vi "ExamplePIDDrive.vi"() -> ()   [LabVIEW 2016]
uses:
  <vilib>/addons/control/pid/pid.llb/PID (DBL).vi
  <vilib>/addons/control/pid/NI_PID_pid.lvlib
panel:
  in  "PID Segments (1-500)":dbl=1.0
  in  "Limit of Orientation Change":dbl=1.0
  in  "Absolute Theta Final":dbl
  in  "Absolute Theta initial":dbl
  in  "Y":dbl[](array[numeric])
  in  "X":dbl[](array[numeric])
  out "output 2":dbl format="%.2f"
  out "output":dbl format="%.2f"
  in  "Steer Range":cluster{"output high":dbl, "output low":dbl}={"output high"=100.0, "output low"=-100.0} {"output low" format="%.2f"; "output high" format="%.2f"}
  in  "PID Steer gains":T1={"proportional gain (Kc)"=1.0, "integral time (Ti, min)"=0.01, "derivative time (Td, min)"=0.0} {"derivative time (Td, min)" format="%.3f"; "integral time (Ti, min)" format="%.3f"; "proportional gain (Kc)" format="%.3f"}
  in  "Speed Range":cluster{"output high":dbl, "output low":dbl}={"output high"=100.0, "output low"=-100.0} {"output low" format="%.2f"; "output high" format="%.2f"}
  in  "PID Speed gains":T1={"proportional gain (Kc)"=1.0, "integral time (Ti, min)"=0.01, "derivative time (Td, min)"=0.0} {"derivative time (Td, min)" format="%.3f"; "integral time (Ti, min)" format="%.3f"; "proportional gain (Kc)" format="%.3f"}
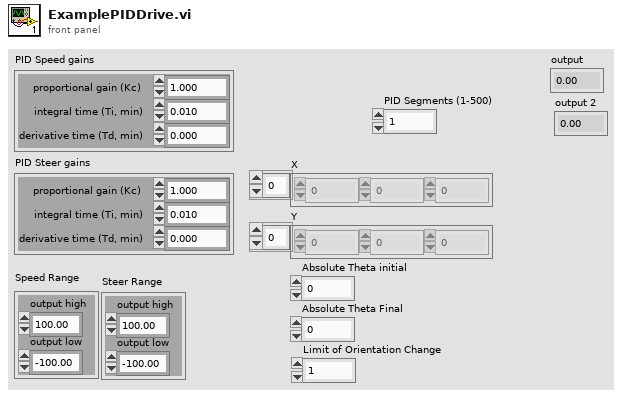
[diagram p1: front panel]
types:
  T1 = cluster{"proportional gain (Kc)":dbl, "integral time (Ti, min)":dbl, "derivative time (Td, min)":dbl}
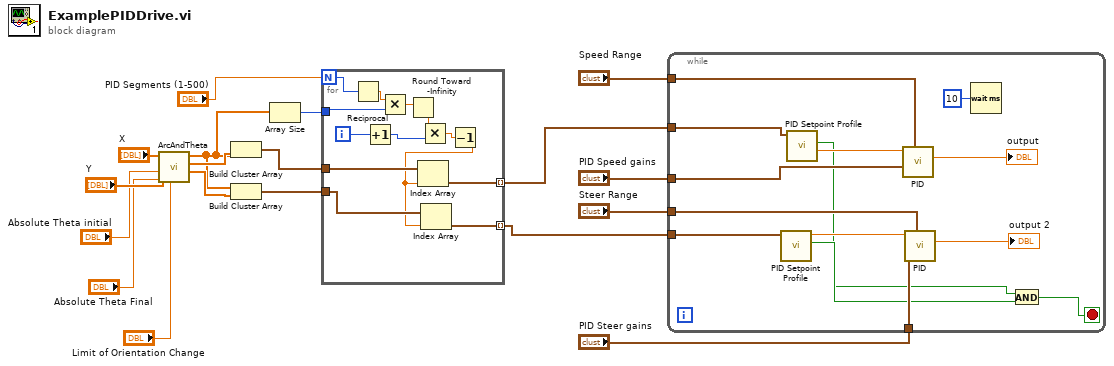
[diagram p0: block diagram]
diagram:
  n1 = call "ArcAndTheta.vi"("Limit of Orientation Change"="Limit of Orientation Change", "Absolute Theta Final"="Absolute Theta Final", "Absolute Theta initial"="Absolute Theta initial", "Y"="Y", "X"="X") -> ("Theta(arc length)"=w17:dbl[], "Arc Length"=w18:dbl[], "TimeStamp"=w10:dbl[])  [unwired: 3 in, 1 out]
  n2 = Build Cluster Array(w10, w18) -> (w8:cluster{dbl, dbl}[])
  n3 = Build Cluster Array(w10, w17) -> (w7:cluster{dbl, dbl}[])
  n4 = Array Size(array=w10) -> (size(s)=w9:i32)
  n5 = for {
    N: "PID Segments (1-500)" -> [w31]
    tunnel: w9 -> [w29]
    tunnel: w8 -> [w23]
    tunnel: w7 -> [w22]
    tunnel: [w20] -> w2 mode=indexing
    tunnel: [w19] -> w1 mode=indexing
    i -> [w27]
    n6 = Reciprocal(x=w31) -> (1/x=w30:dbl)
    n7 = Increment(x=w27) -> (x+1=w26:i32)
    n8 = Multiply(x=w30, y=w29) -> (x*y=w28:dbl)
    n9 = Round Toward -Infinity(1:w28) -> (0:w25:dbl)
    n10 = Multiply(x=w25, y=w26) -> (x*y=w24:dbl)
    n11 = Decrement(x=w24) -> (x-1=w21:dbl)
    n12 = Index Array(array=w23, index=w21) -> (element=w20:cluster{dbl, dbl})
    n13 = Index Array(array=w22, index=w21) -> (element=w19:cluster{dbl, dbl})
  }
  n14 = while {
    tunnel: "PID Speed gains" -> [w45]
    tunnel: "Speed Range" -> [w44]
    tunnel: "PID Steer gains" -> [w43]
    tunnel: "Steer Range" -> [w42]
    tunnel: w2 -> [w33]
    tunnel: w1 -> [w32]
    stop <- w37 stop-if-true
    n15 = call <vilib>:"PID Setpoint Profile.vi"("setpoint profile"=w32) -> ("profile complete?"=w39:bool, "setpoint"=w41:dbl)  [unwired: 5 in, 2 out]
    n16 = call <vilib>:"PID Setpoint Profile.vi"("setpoint profile"=w33) -> ("profile complete?"=w38:bool, "setpoint"=w40:dbl)  [unwired: 5 in, 2 out]
    n17 = call-poly <vilib>:"PID.vi"("output range"=w44, "PID gains"=w45, "setpoint"=w40) -> ("output"=→"output":dbl)  [unwired: 7 in, 1 out]
    n18 = call-poly <vilib>:"PID.vi"("output range"=w42, "PID gains"=w43, "setpoint"=w41) -> ("output"=→"output 2":dbl)  [unwired: 7 in, 1 out]
    n19 = Wait (ms)(milliseconds to wait=u32 10) -> ()  [unwired: 1 out]
    n20 = And(x=w38, y=w39) -> (x .and. y?=w37:bool)
  }
